vi "svx_Waterfall Frequency Cursor.vi"(0 "cursors":T8[](array[typedef]), 1 "waterfall data":T7, 2 "frequency (60 Hz)":dbl=60.0 min=0.0, 3 "speeds [RPM]":dbl[](array[numeric]), 4 "spectrum info":T1={"channel name"="", "description"="", "x-axis units"=0, "spectral info"={"spectrum type"=enum."Power [Magnitude^2]", "linear/dB"=enum."linear", "window"=0, "window size"=0, "FFT size"=0}, "engineering units"=0, "custom label"="", "dB reference [EU]"=0.0, "peak units"=enum."rms", "weighting filter"=0, "spectral density?"=FALSE, "unit label"="", "spectrum skewed?"=FALSE, "complimentary spectrum units"=enum."none"} {"x-axis units" items=["Time (s)"=0, "Frequency-CB (Hz)"=1, "Frequency-CPB (Hz)"=1248, "Frequency-Arbitrary (Hz)"=2357, "Quefrency (s)"=2, "Revolutions (rev)"=3, "Order"=4, "Speed (RPM)"=11, "Speed (rad/s)"=21, "Index"=65535]; "weighting filter" items=["Linear", "A-weighting", "B-weighting", "C-weighting", "ITU-R 468-4", "Dolby", "CCITT", "C-message", "Wb", "Wc", "Wd", "We", "Wf", "Wh", "Wj", "Wk", "Wm", "AES17 20 kHz lowpass", "AES17 40 kHz lowpass", "AES17 20 kHz highpass", "AES17 40 kHz highpass"]; "dB reference [EU]" format="%.2f"; "engineering units" items=["custom..."=0, "V"=1, "A"=21, "C"=30, "pC"=31, "s"=32, "-"=29, "Pa"=2, "N"=20, "g"=3, "m/s^2"=4, "m/s"=5, "m"=6, "mm/s"=12, "mm"=13, "micron/s"=14, "micron"=15, "in/s^2"=7, "in/s"=8, "in"=9, "mil/s"=10, "mil"=11, "rad/s^2"=16, "rad/s"=17, "rad"=18, "deg/s^2"=26, "deg/s"=27, "deg"=28, "RPM"=22, "cycle/s^2"=23, "Hz"=24, "cycle"=25, "strain"=19]; "spectral info"."window" items=["None "=0, "Hanning"=1, "Hamming"=2, "Blackman-Harris"=3, "Exact Blackman"=4, "Blackman"=5, "Flat Top"=6, "4 Term B-Harris "=7, "7 Term B-Harris"=8, "Low Sidelobe"=9, "Force - Exponential"=10, "Gaussian"=62]}, 5 "error in (no error)":errorcluster, 6 "coercion (nearest)":T9(ring)) -> (14 "appended cursors":T8[](array[typedef]), 15 "duplicate waterfall data":T7, 16 "cursor data":cluster{"X":dbl, "Y":dbl, "Z":dbl}[](array[cluster]), 17 "cursor index":i32, 18 "duplicate spectrum info":T1={"channel name"="", "description"="", "x-axis units"=0, "spectral info"={"spectrum type"=enum."Power [Magnitude^2]", "linear/dB"=enum."linear", "window"=0, "window size"=0, "FFT size"=0}, "engineering units"=0, "custom label"="", "dB reference [EU]"=0.0, "peak units"=enum."rms", "weighting filter"=0, "spectral density?"=FALSE, "unit label"="", "spectrum skewed?"=FALSE, "complimentary spectrum units"=enum."none"} {"x-axis units" items=["Time (s)"=0, "Frequency-CB (Hz)"=1, "Frequency-CPB (Hz)"=1248, "Frequency-Arbitrary (Hz)"=2357, "Quefrency (s)"=2, "Revolutions (rev)"=3, "Order"=4, "Speed (RPM)"=11, "Speed (rad/s)"=21, "Index"=65535]; "weighting filter" items=["Linear", "A-weighting", "B-weighting", "C-weighting", "ITU-R 468-4", "Dolby", "CCITT", "C-message", "Wb", "Wc", "Wd", "We", "Wf", "Wh", "Wj", "Wk", "Wm", "AES17 20 kHz lowpass", "AES17 40 kHz lowpass", "AES17 20 kHz highpass", "AES17 40 kHz highpass"]; "dB reference [EU]" format="%.2f"; "engineering units" items=["custom..."=0, "V"=1, "A"=21, "C"=30, "pC"=31, "s"=32, "-"=29, "Pa"=2, "N"=20, "g"=3, "m/s^2"=4, "m/s"=5, "m"=6, "mm/s"=12, "mm"=13, "micron/s"=14, "micron"=15, "in/s^2"=7, "in/s"=8, "in"=9, "mil/s"=10, "mil"=11, "rad/s^2"=16, "rad/s"=17, "rad"=18, "deg/s^2"=26, "deg/s"=27, "deg"=28, "RPM"=22, "cycle/s^2"=23, "Hz"=24, "cycle"=25, "strain"=19]; "spectral info"."window" items=["None "=0, "Hanning"=1, "Hamming"=2, "Blackman-Harris"=3, "Exact Blackman"=4, "Blackman"=5, "Flat Top"=6, "4 Term B-Harris "=7, "7 Term B-Harris"=8, "Low Sidelobe"=9, "Force - Exponential"=10, "Gaussian"=62]}, 19 "error out":errorcluster)   [LabVIEW 2017]
doc: "Creates either a frequency or order cursor that can be plotted on a waterfall graph. Use the waterfall graph property node \"lines\" to draw the cursor on the graph."
uses:
  <vilib>/addons/_NISVFA/_Shared subVIs/Controls/svc_Spectrum Info.ctl
  <vilib>/addons/_NISVFA/_Shared subVIs/Controls/svc_X-Axis Units.ctl
  <vilib>/addons/_NISVFA/_Shared subVIs/Controls/svc_Spectrum Type.ctl
  <vilib>/addons/_NISVFA/_Shared subVIs/Controls/svc_Engineering Units Text Ring.ctl
  <vilib>/addons/_NISVFA/_Shared subVIs/Controls/svc_Weighting Filter Text Ring.ctl
  <vilib>/addons/_NISVFA/_Shared subVIs/Controls/svc_Complimentary Spectrum Units.ctl
  <vilib>/addons/_NISVFA/_Shared subVIs/Controls/svc_Cluster of Array of Cluster of XYZ.ctl
  <vilib>/addons/_XControls/Utility/subVIs/svx_Waterfall Add Cursor.vi
  <vilib>/addons/_NISVFA/_Spectrum Processing/SVFA Get Waterfall Value (Scalar X).vi
  <vilib>/addons/_NISVFA/_Spectrum Processing/SVFA Get Waterfall Value (Array X).vi
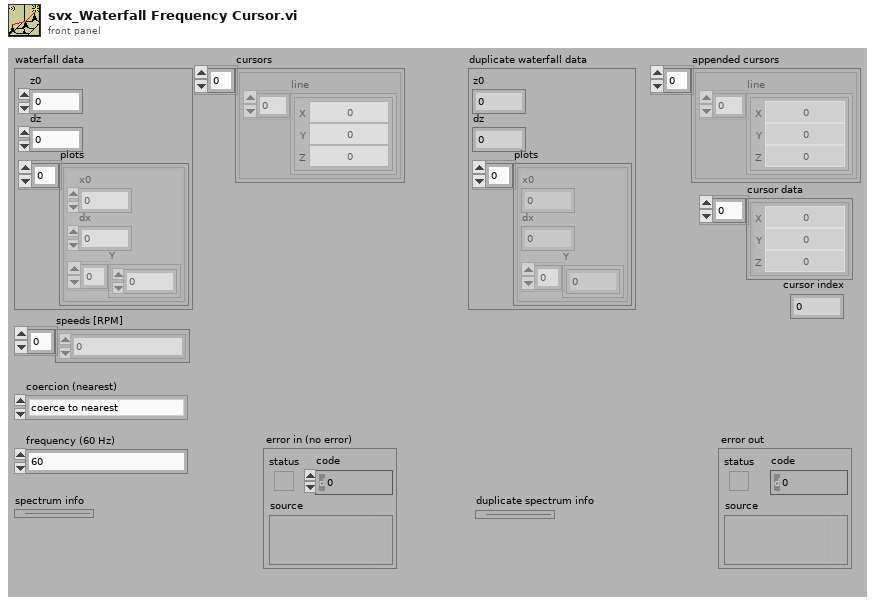
[diagram p1: front panel]
types:
  T1 = typedef "svc_Spectrum Info.ctl" = cluster{"channel name":string, "description":string, "x-axis units":T2, "spectral info":cluster{"spectrum type":T3, "linear/dB":enum16{"linear", "dB"}, "window":u16, "window size":i32, "FFT size":i32}, "engineering units":T4, "custom label":string, "dB reference [EU]":dbl, "peak units":enum16{"rms", "peak", "peak-peak"}, "weighting filter":T5, "spectral density?":bool, "unit label":string, "spectrum skewed?":bool, "complimentary spectrum units":T6}
  T2 = typedef "svc_X-Axis Units.ctl" = u16
  T3 = typedef "svc_Spectrum Type.ctl" = enum16{"FFT Spectrum [complex]", "Amplitude [Magnitude]", "Power [Magnitude^2]", "Cross Spectrum [complex]", "Frequency Response [Complex]"}
  T4 = typedef "svc_Engineering Units Text Ring.ctl" = u16
  T5 = typedef "svc_Weighting Filter Text Ring.ctl" = u16
  T6 = typedef "svc_Complimentary Spectrum Units.ctl" = enum16{"none", "radians", "degrees", "cycles", "imaginary"}
  T7 = cluster{"z0":dbl, "dz":dbl, "plots":cluster{"x0":dbl, "dx":dbl, "Y":dbl[]}[]}
  T8 = typedef "svc_Cluster of Array of Cluster of XYZ.ctl" = cluster{"line":cluster{"X":dbl, "Y":dbl, "Z":dbl}[]}
  T9 = enum16{"coerce to nearest", "coerce to next highest", "coerce to next lowest", "interpolate"}
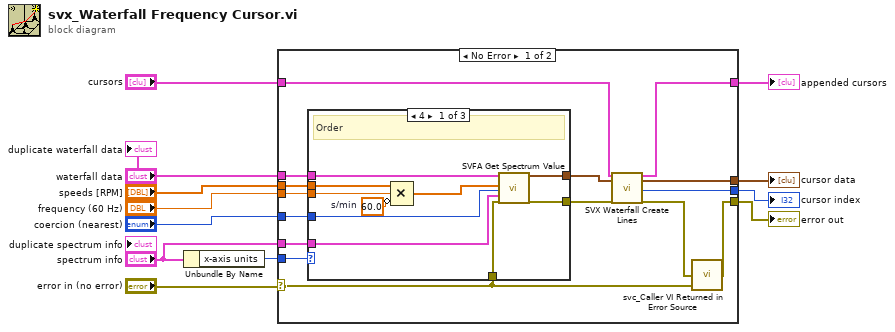
[diagram p0: block diagram]
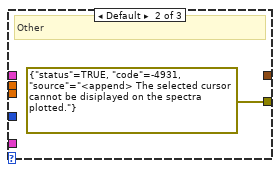
[diagram p2: hidden frame]
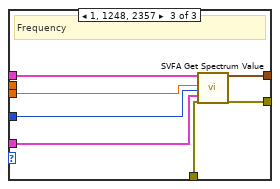
[diagram p3: hidden frame]
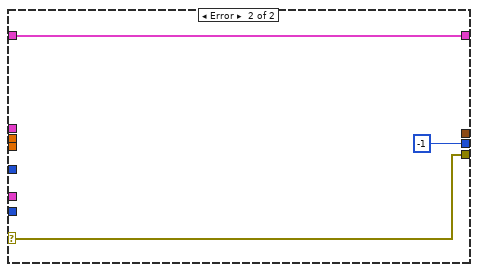
[diagram p4: hidden frame]
diagram:
  n1 = Unbundle By Name("spectrum info") -> ("x-axis units"=w8:T2)
  n2 = case shown="No Error" "error in (no error)" {
    selector: "error in (no error)" -> [w15 w48]
    tunnel: [w22 w47] -> w7
    tunnel: "spectrum info" -> [w27 _]
    tunnel: "speeds [RPM]" -> [w26 _]
    tunnel: "coercion (nearest)" -> [w25 _]
    tunnel: [w13 w48] -> w11
    tunnel: w8 -> [w24 _]
    tunnel: "cursors" -> [w23 w47]
    tunnel: [w21 _] -> w4
    tunnel: [w20 -1] -> w5
    tunnel: "waterfall data" -> [w19 _]
    tunnel: "frequency (60 Hz)" -> [w16 _]
    frame No Error {
      n3 = case shown="4" w24 {
        tunnel: [w36 _ w44] -> w18
        tunnel: w16 -> [w30 _ w43]
        tunnel: w27 -> [w33 _ w41]
        tunnel: w26 -> [w31 _ _]
        tunnel: w25 -> [w34 _ w42]
        tunnel: [w35 errorcluster {"status"=TRUE, "code"=-4931, "source"="<append> The selected cursor cannot be disiplayed on the spectra plotted."} ("error IO") w40] -> w17
        tunnel: w19 -> [w37 _ w45]
        tunnel: w15 -> [w28 _ w39]
        frame 4 {
          w32 = 60.0  # s/min
          # "Order"
          n4 = Compound Arithmetic op=MULTIPLY(w31, w30, invert w32) -> (w29:dbl[])
          n5 = call-poly <vilib>:"SVFA Get Spectrum Value.vi"("waterfall data"=w37, "x values"=w29, "coercion (nearest)"=w34, "spectrum info"=w33, "error in"=w28) -> ("waterfall values"=w36:cluster{"X":dbl, "Y":dbl, "Z":dbl}[], "error out"=w35:errorcluster)  [unwired: 13 in]
        }
        frame Default {
          # "Other"
        }
        frame 1, 1248, 2357 {
          # "Frequency"
          n6 = call-poly <vilib>:"SVFA Get Spectrum Value.vi"("waterfall data"=w45, "x value (1000)"=w43, "coercion (nearest)"=w42, "spectrum info"=w41, "error in"=w39) -> ("waterfall values"=w44:cluster{"X":dbl, "Y":dbl, "Z":dbl}[], "error out"=w40:errorcluster)  [unwired: 13 in]
        }
      }
      n7 = call-poly <vilib>:"SVX Waterfall Create Lines.vi"("cursors"=w23, "cursor points"=w18, "error in (no error)"=w17) -> ("appended cursors"=w22:T8[], "duplicate cursor points"=w21:cluster{"X":dbl, "Y":dbl, "Z":dbl}[], "cursor index"=w20:i32, "error out"=w14:errorcluster)  [unwired: 13 in]
      n8 = call <vilib>:"svc_Caller VI Returned in Error Source.vi"("warning input to caller"=w15, "error in (no error)"=w14) -> ("error out"=w13:errorcluster)  [unwired: 3 in]
    }
    frame Error {
    }
  }
  "error out" <- w11
  "appended cursors" <- w7
  "cursor index" <- w5
  "cursor data" <- w4
  "duplicate waterfall data" <- "waterfall data"
  "duplicate spectrum info" <- "spectrum info"
